vi "Program26.vi"() -> ()   [LabVIEW 2020]
panel:
  in  "Tekst":string
  out "Nowe Dane 2":T1
  out "Nowe Dane":T1
  in  "Dane wejsciowe":T1
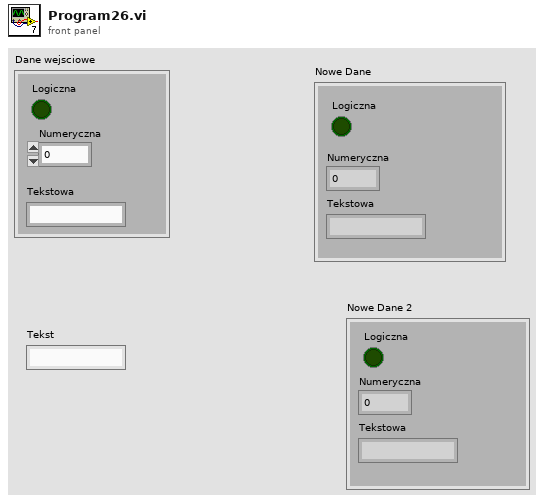
[diagram p1: front panel]
types:
  T1 = cluster{"Logiczna":bool, "Numeryczna":dbl, "Tekstowa":string}
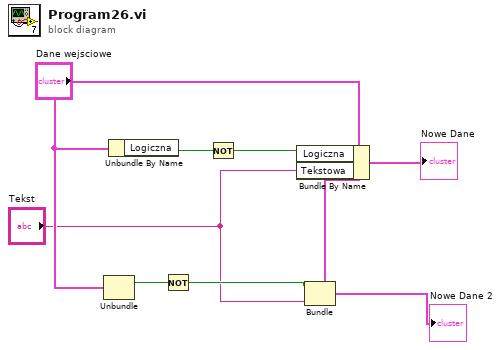
[diagram p0: block diagram]
diagram:
  n1 = Unbundle("Dane wejsciowe") -> ("Logiczna"=w3:bool)  [unwired: 2 out]
  n2 = Unbundle By Name("Dane wejsciowe") -> ("Logiczna"=w8:bool)
  n3 = Not(x=w3) -> (.not. x?=w2:bool)
  n4 = Not(x=w8) -> (.not. x?=w7:bool)
  n5 = Bundle By Name(cluster="Dane wejsciowe", "Logiczna"=w7, "Tekstowa"="Tekst") -> (→"Nowe Dane":T1)
  n6 = Bundle(cluster="Dane wejsciowe", "Logiczna"=w2, "Tekstowa"="Tekst") -> (→"Nowe Dane 2":T1)  [unwired: 1 in]
